vi "G-Vibro.vi"() -> ()   [LabVIEW 2016]
uses:
  <instrlib>/niScope/Controls/niScope trigger source.ctl
  <vilib>/Motion/FlexMotion/CustomControls/CustomControls.llb/AxisOrVectorSpace To Configure.flx
  <vilib>/Motion/FlexMotion/CustomControls/CustomControls.llb/AxisOrVectorSpaceControl To Control.flx
  <vilib>/event_ctls.llb/eventvkey.ctl
  <vilib>/Utility/file.llb/Write To Spreadsheet File (DBL).vi
  <vilib>/Motion/FlexMotion/FunctionsVIs/StartStopMotion.llb/Start Motion (8 axes).flx
  <vilib>/Motion/FlexMotion/FunctionsVIs/StartStopMotion.llb/Stop Motion (8 axes).flx
panel:
  out "Aceleration (pulse/s2)":i32
  out "Velocity (pulse/s)":i32
  in  "Power spectrum unit":string(combo)
  in  "Time unit":string(combo)
  in  "Highpass cut (kHz)":dbl=100.0
  in  "Center positioned":bool=TRUE
  out "Time (us)":dbl=-1000000.0
  out "Distance (mm)":dbl=-1480000.0
  out "Peak to peak":dbl
  in  "Lowpass filter":bool
  in  "Lowpass cut (kHz)":dbl=100.0
  out "Frequency Graph":cluster{"f0":dbl, "df":dbl, "magnitude":dbl[]}(graph)={"f0"=0.0, "df"=inf, "magnitude"=[]}
  out "z":dbl
  out "y":dbl=6.0
  out "x":dbl
  in  "Pulses":i32=20 min=1 max=100 step=1
  in  "Save to...":path=path "C:/Users/Vibro-PC/Desktop/Codigos em Labview/Data"
  in  "stop":bool
  in  "dz (mm)":dbl=1.0
  in  "Nz":i32=1 min=1 max=10000 step=1
  in  "dy (mm)":dbl=0.25
  in  "Ny":i32=56 min=1 max=10000 step=1
  in  "dx (mm)":dbl=0.25
  in  "Nx":i32=56 min=1 max=10000 step=1
  in  "Aceleration (mm/s2)":dbl=1000.0 min=50.0 max=1250.0 step=10.0
  out "Time Graph":waveform(dbl)(graph)={"t0"=timestamp(0 s since 1904-01-01), "dt"=1000000.0, "Y"=[]}
  in  "Enable Oscilloscope":bool
  in  "Move (mm)":dbl=6.0
  in  "Move Far":bool
  in  "Move Close":bool
  in  "Move Down":bool
  in  "Move Right":bool
  in  "Move Left":bool
  in  "Move Up":bool
  in  "Jog Far":bool
  in  "Jog Close":bool
  in  "Jog Down":bool
  in  "Jog Right":bool
  in  "Jog Left":bool
  in  "Jog Up":bool
  in  "Multiplier":dbl(slide)=0.10000000000000014 min=0.1 max=1.001 step=0.1 scale=0.1..1.0
  in  "Velocity (mm/s)":dbl=20.0 min=1.0 max=200.0 step=1.0
  in  "trigger level":dbl=2.0 caption="Level (V)" min=0.2 max=10.0 step=0.2 format="%.2f"
  in  "trigger source":T1="VAL_EXTERNAL" caption="Source"
  in  "Time (us)":dbl=2000.0 min=1.0 max=10000.0 step=1.0
  in  "Sample rate (MHz)":dbl=1.0 min=0.0 max=150.0 step=0.1 format="%.2f"
  in  "vertical offset":dbl caption="Offset (V)" min=-10.0 max=10.0 step=0.2 format="%.4f"
  in  "vertical range":dbl=2.0 caption="Vertical range (V)" min=0.0 max=20.0 format="%.2f"
  in  "# Channel":i32 min=0 max=1 step=1
  in  "Ajust Axis":bool
  in  "resource name":refnum<k15>="Dev1" caption="Source"
  # "Oscilloscope"
  # "Axis Stage"
  # "Channel Control"
  # "Temporal Control"
  # "Trigger Control"
  # "Status"
  # "Jog"
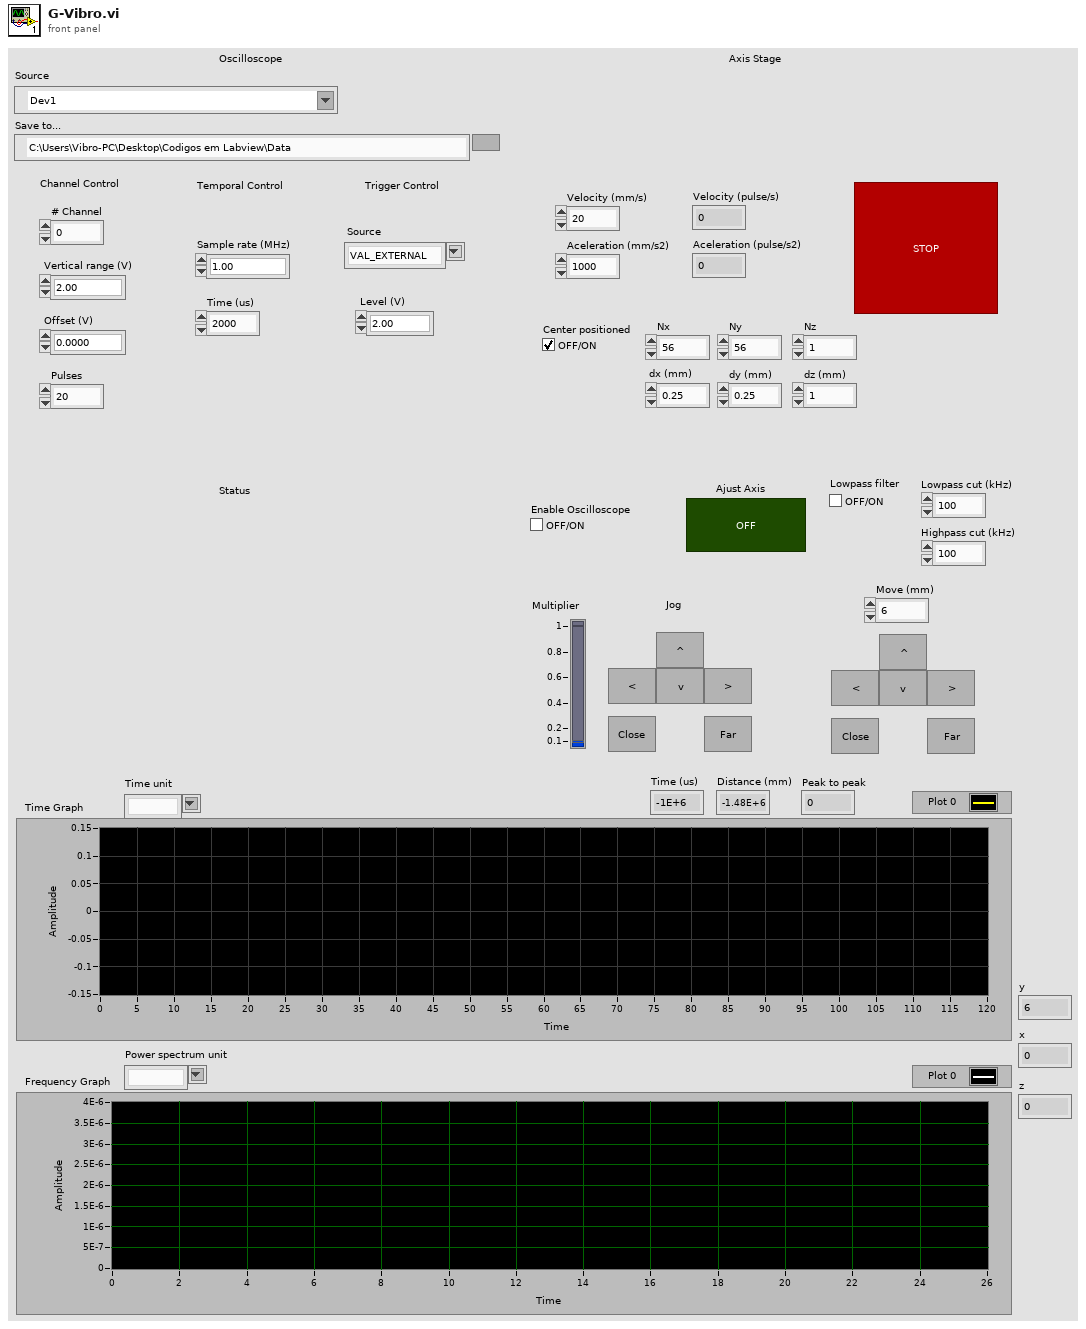
[diagram p1: front panel]
types:
  T1 = typedef "niScope trigger source.ctl" = string
  T2 = typedef "Board Id" = u8
  T3 = typedef "Bd Id Out" = u8
  T4 = enum16{"Absolute Position", "Relative Position", "Velocity", "Relative to Cap Pos", "Modulus Position", "Absolute Contouring", "Relative Contouring"}
  T5 = typedef "eventvkey.ctl" = enum16{"ASCII", "Enter", "Return", "Shift", "Ctrl", "Alt", "Cmd", "Opt", "Caps", "NumLock", "Clear", "Break", "Up", "Down", "Left", "Right", "Insert", "Delete", "Home", "End", "PageUp", "PageDown", "Escape", "Help", "Pause", "ScrollLock", "F1", "F2", "F3", "F4", "F5", "F6", "F7", "F8", "F9", "F10", "F11", "F12", "F13", "F14", "F15", "F16", "F17", "F18", "F19", "F20", "F21", "F22", "F23", "F24", "Play", "VolumeUp", "VolumeDown", "Mute", "Two Byte Char"}
  T6 = typedef "AxisOrVectorSpace To Configure.flx" = u16
  T7 = typedef "AxisOrVectorSpaceControl To Control.flx" = u16
  T8 = typedef "Resource Out (Enum).flx" = u16
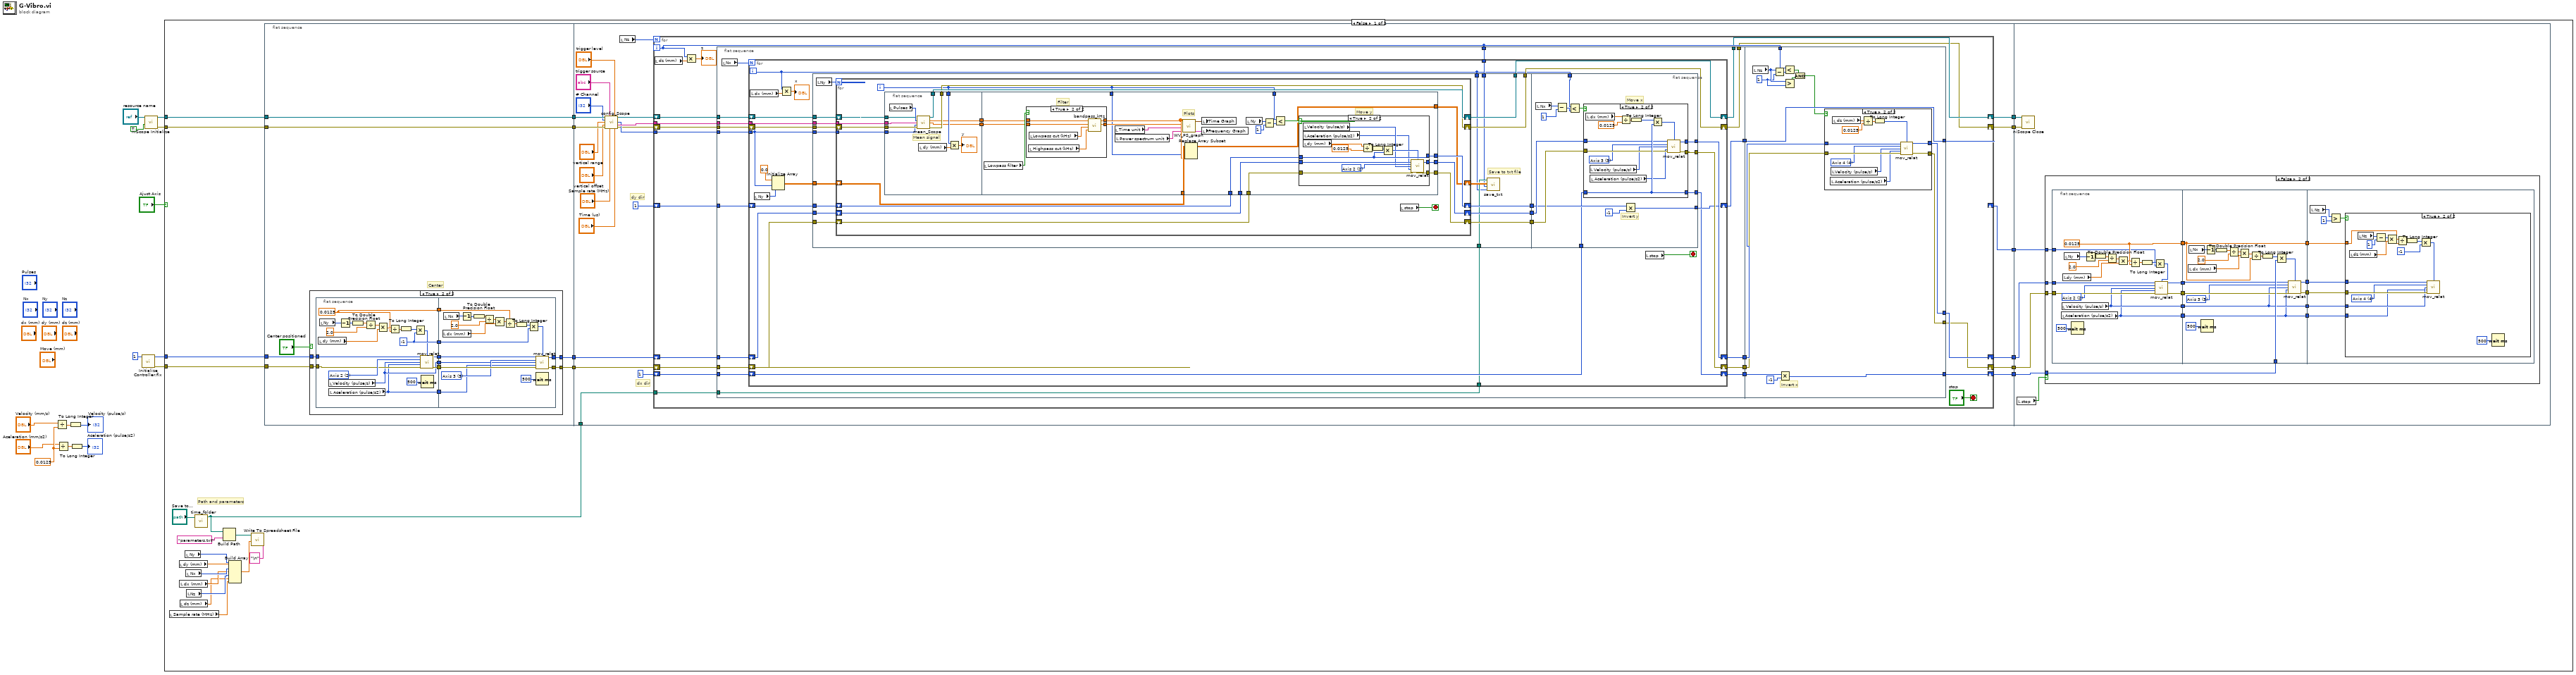
[diagram p0: block diagram]
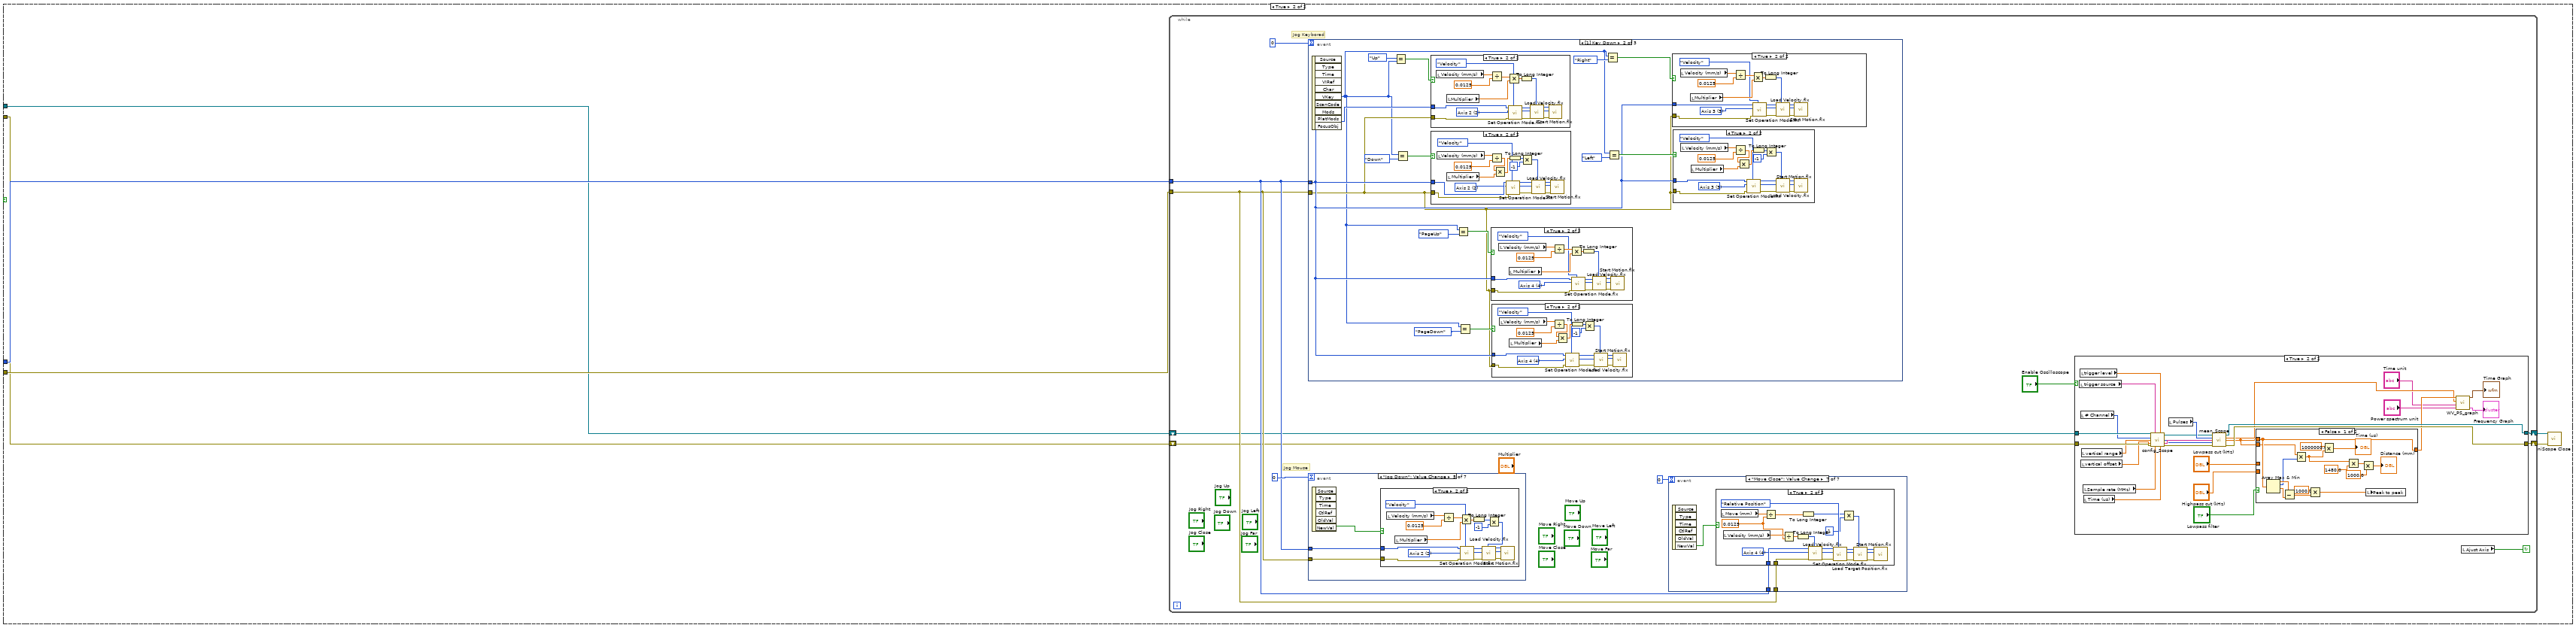
[diagram p9: hidden frame]
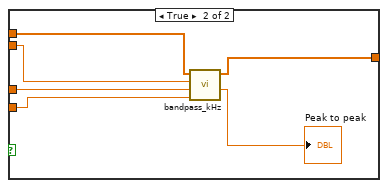
[diagram p11: hidden frame]
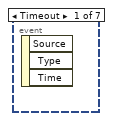
[diagram p12: hidden frame]
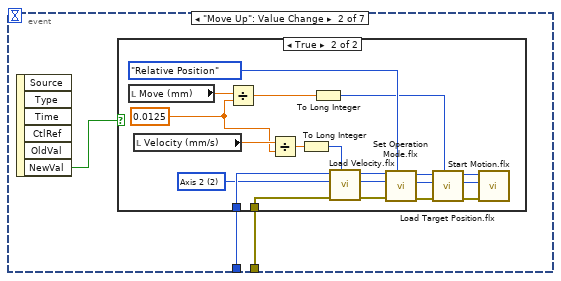
[diagram p13: hidden frame]
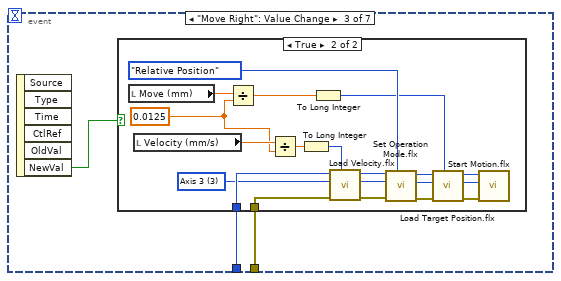
[diagram p15: hidden frame]
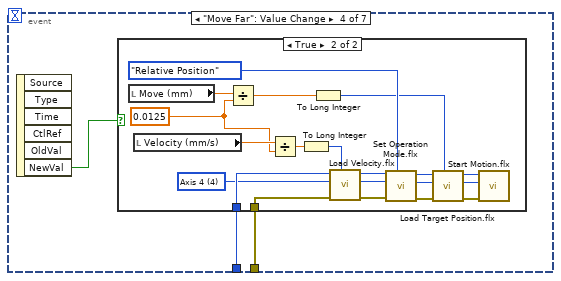
[diagram p17: hidden frame]
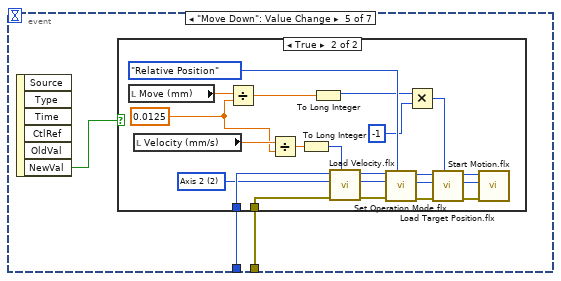
[diagram p19: hidden frame]
diagram:
  w6 = 0.0125
  n1 = Divide(x="Velocity (mm/s)", y=w6) -> (x/y=w4:dbl)
  n2 = Divide(x="Aceleration (mm/s2)", y=w6) -> (x/y=w3:dbl)
  n3 = To Long Integer(number=w4) -> (32bit integer=→"Velocity (pulse/s)":i32)
  n4 = To Long Integer(number=w3) -> (32bit integer=→"Aceleration (pulse/s2)":i32)
  n5 = call <vilib>:"Initialize Controller.flx"("Board ID"=T2 1) -> ("error out"=w9:errorcluster, "Bd ID Out"=w10:T3)  [unwired: 7 in]
  n6 = call <instrlib>:"niScope Initialize.vi"("resource name"="resource name", "reset device"=TRUE) -> ("instrument handle"=w13:refnum<k15>, "error out"=w12:errorcluster)  [unwired: 12 in]
  n7 = case shown="False" "Ajust Axis" {
    tunnel: w13 -> [w42 w432]
    tunnel: w12 -> [w41 w433]
    tunnel: w10 -> [w40 w435]
    tunnel: w9 -> [w39 w434]
    frame False {
      # "Path and parameters"
      n8 = local read "Sample rate (MHz)"() -> (w18:dbl)
      n9 = local read "dy (mm)"() -> (w23:dbl)
      n10 = local read "dx (mm)"() -> (w21:dbl)
      n11 = local read "dz (mm)"() -> (w19:dbl)
      n12 = local read "Ny"() -> (w24:i32)
      n13 = local read "Nx"() -> (w22:i32)
      n14 = local read "Nz"() -> (w20:i32)
      n15 = call "time_folder.vi"("base path"="Save to...") -> ("folder path"=w16:path)  [unwired: 9 in, 1 out]
      n16 = Build Path(base path=w16, name or relative path="parameters.txt") -> (appended path=w27:path)
      n17 = Build Array(w24, w23, w22, w21, w20, w19, w18) -> (w25:dbl[])
      n18 = call-poly <vilib>:"Write To Spreadsheet File.vi"("delimiter (\\t)"="\n", "1D data"=w25, "file path (dialog if empty)"=w27) -> ()  [unwired: 5 in, 1 out]
      n19 = flat-sequence {
        tunnel: w39 -> [w46]
        tunnel: w40 -> [w47]
        tunnel: w41 -> [w48]
        tunnel: w42 -> [w49]
        tunnel: [w49] -> w38
        tunnel: [w48] -> w37
        tunnel: [w45] -> w36
        tunnel: [w44] -> w35
        tunnel: w38 -> [w112]
        tunnel: w37 -> [w111]
        tunnel: w36 -> [w125]
        tunnel: w35 -> [w124]
        tunnel: [w121] -> w34
        tunnel: [w120] -> w33
        tunnel: [w119] -> w32
        tunnel: [w118] -> w31
        tunnel: [w117] -> w30
        tunnel: [w116] -> w29
        tunnel: w16 -> [w115]
        tunnel: w34 -> [w349]
        tunnel: w33 -> [w348]
        tunnel: w32 -> [w351]
        tunnel: w31 -> [w350]
        tunnel: w30 -> [w347]
        tunnel: w29 -> [w346]
        frame #0 {
          # "Center"
          n20 = case shown="True" "Center positioned" {
            tunnel: w47 -> [w51 w59]
            tunnel: w46 -> [w50 w58]
            tunnel: [w51 w53] -> w45
            tunnel: [w50 w52] -> w44
            frame False {
            }
            frame True {
              n21 = flat-sequence {
                tunnel: w59 -> [w67]
                tunnel: w58 -> [w66]
                tunnel: [w77] -> w61
                tunnel: [w75] -> w60
                tunnel: [w65] -> w57
                tunnel: [w64] -> w56
                tunnel: [w63] -> w55
                tunnel: [w62] -> w54
                tunnel: w61 -> [w97]
                tunnel: w60 -> [w95]
                tunnel: w57 -> [w89]
                tunnel: w56 -> [w88]
                tunnel: w55 -> [w86]
                tunnel: w54 -> [w85]
                tunnel: [w83] -> w53
                tunnel: [w82] -> w52
                frame #0 {
                  w75 = -1 ("y")
                  w77 = 0.0125
                  w68 = T6 2 items=["Axis 1"=1, "Axis 2"=2, "Axis 3"=3, "Axis 4"=4, "Axis 5"=5, "Axis 6"=6, "Axis 7"=7, "Axis 8"=8, "Vector Space 1"=17, "Vector Space 2"=18, "Vector Space 3"=19, "Vector Space 4"=20] ("Axis or Vector Space")
                  n22 = local read "dy (mm)"() -> (w80:dbl)
                  n23 = local read "Ny"() -> (w73:i32)
                  n24 = local read "Velocity (pulse/s)"() -> (w63:i32)
                  n25 = local read "Aceleration (pulse/s2)"() -> (w62:i32)
                  n26 = Decrement(x=w73) -> (x-1=w71:i32)
                  n27 = To Double Precision Float(number=w71) -> (double precision float=w72:dbl)
                  n28 = Divide(x=w72, y=2.0) -> (x/y=w81:dbl)
                  n29 = Multiply(x=w81, y=w80) -> (x*y=w79:dbl)
                  n30 = Divide(x=w79, y=w77) -> (x/y=w78:dbl)
                  n31 = To Long Integer(number=w78) -> (32bit integer=w76:i32)
                  n32 = Multiply(x=w76, y=w75) -> (x*y=w69:i32)
                  n33 = call "mov_relat.vi"("Board ID"=w67, "Target Position (0)"=w69, "Axis or Vector Space"=w68, "Velocity (10000)"=w63, "Acceleration (100000)"=w62, "error in (no error)"=w66) -> ("Bd ID Out"=w65:T3, "error out"=w64:errorcluster)  [unwired: 8 in]
                  n34 = Wait (ms)(milliseconds to wait=u32 500) -> ()  [unwired: 1 out]
                }
                frame #1 {
                  w87 = T6 3 items=["Axis 1"=1, "Axis 2"=2, "Axis 3"=3, "Axis 4"=4, "Axis 5"=5, "Axis 6"=6, "Axis 7"=7, "Axis 8"=8, "Vector Space 1"=17, "Vector Space 2"=18, "Vector Space 3"=19, "Vector Space 4"=20] ("Axis or Vector Space")
                  n35 = local read "dx (mm)"() -> (w98:dbl)
                  n36 = local read "Nx"() -> (w93:i32)
                  n37 = Decrement(x=w93) -> (x-1=w91:i32)
                  n38 = To Double Precision Float(number=w91) -> (double precision float=w92:dbl)
                  n39 = Divide(x=w92, y=2.0) -> (x/y=w101:dbl)
                  n40 = Multiply(x=w101, y=w98) -> (x*y=w100:dbl)
                  n41 = Divide(x=w100, y=w97) -> (x/y=w99:dbl)
                  n42 = To Long Integer(number=w99) -> (32bit integer=w96:i32)
                  n43 = Multiply(x=w96, y=w95) -> (x*y=w84:i32)
                  n44 = Wait (ms)(milliseconds to wait=u32 500) -> ()  [unwired: 1 out]
                  n45 = call "mov_relat.vi"("Board ID"=w89, "Target Position (0)"=w84, "Axis or Vector Space"=w87, "Velocity (10000)"=w86, "Acceleration (100000)"=w85, "error in (no error)"=w88) -> ("Bd ID Out"=w83:T3, "error out"=w82:errorcluster)  [unwired: 8 in]
                }
              }
            }
          }
        }
        frame #1 {
          # "dx dir"
          # "dy dir"
          n46 = call "config_Scope.vi"("instrument handle"=w112, "trigger source"="trigger source", "trigger level"="trigger level", "Channel"="# Channel", "vertical range"="vertical range", "vertical offset"="vertical offset", "error in"=w111, "Frequency(MHz)"="Sample rate (MHz)", "Time(us)"="Time (us)") -> ("instrument handle out"=w103:refnum<k15>, "Record length"=w113:i32, "Channel out"=w114:string, "error out"=w102:errorcluster)  [unwired: 3 in]
          n47 = local read "Nz"() -> (w126:i32)
          n48 = for {
            N: w126 -> [_]
            tunnel: w114 -> [w146]
            shift-right: [w127] -> w118
            shift-left: w102 -> [w147]
            shift-right: [w128] -> w119
            shift-left: w103 -> [w148]
            shift-right: [w135] -> w121
            shift-left: w125 -> [w145]
            shift-right: [w134] -> w120
            shift-left: w124 -> [w144]
            shift-right: [w142] -> w117
            shift-left: 1 -> [w143]
            shift-right: [w136] -> w116
            shift-left: 1 -> [w141]
            tunnel: w113 -> [w133]
            tunnel: w115 -> [w132]
            i -> [w129]
            stop <- "stop" stop-if-true
            n49 = local read "dz (mm)"() -> (w130:dbl)
            n50 = Multiply(x=w129, y=w130) -> (x*y=→"z":dbl)
            n51 = flat-sequence {
              tunnel: w148 -> [w165]
              tunnel: w147 -> [w164]
              tunnel: w146 -> [w163]
              tunnel: w145 -> [w162]
              tunnel: w144 -> [w161]
              tunnel: w143 -> [w158]
              tunnel: w141 -> [w156]
              tunnel: [w160] -> w140
              tunnel: [w159] -> w139
              tunnel: [w157] -> w138
              tunnel: [w155] -> w137
              tunnel: w133 -> [w154]
              tunnel: w132 -> [w153]
              tunnel: w129 -> [w152]
              tunnel: [w151] -> w128
              tunnel: [w150] -> w127
              tunnel: [w328] -> w136
              tunnel: [w331] -> w142
              tunnel: w140 -> [w320]
              tunnel: w139 -> [w319]
              tunnel: w138 -> [w331]
              tunnel: w137 -> [w329]
              tunnel: w129 -> [w326]
              tunnel: [w318] -> w135
              tunnel: [w317] -> w134
              frame #0 {
                n52 = local read "Nx"() -> (w166:i32)
                n53 = for {
                  N: w166 -> [_]
                  shift-right: [w184] -> w151
                  shift-left: w165 -> [w191]
                  tunnel: w163 -> [w189]
                  shift-right: [w183] -> w150
                  shift-left: w164 -> [w190]
                  shift-right: [w182] -> w160
                  shift-left: w162 -> [w188]
                  shift-right: [w181] -> w159
                  shift-left: w161 -> [w187]
                  shift-right: [w178] -> w157
                  shift-left: w158 -> [w180]
                  shift-right: [w176] -> w155
                  shift-left: w156 -> [w177]
                  tunnel: w154 -> [w171]
                  tunnel: w153 -> [w167]
                  tunnel: w152 -> [w172]
                  i -> [w168]
                  stop <- w192 stop-if-true
                  n54 = local read "dx (mm)"() -> (w170:dbl)
                  n55 = local read "Ny"() -> (w174:i32)
                  n56 = Initialize Array(0.0 ("element"), w171, w174) -> (w173:dbl[][])
                  n57 = Multiply(x=w168, y=w170) -> (x*y=→"x":dbl)
                  n58 = flat-sequence {
                    tunnel: w191 -> [w209]
                    tunnel: w190 -> [w208]
                    tunnel: w189 -> [w207]
                    tunnel: w188 -> [w206]
                    tunnel: w187 -> [w205]
                    tunnel: [w204] -> w186
                    tunnel: [w203] -> w185
                    tunnel: [w202] -> w184
                    tunnel: [w201] -> w183
                    tunnel: w180 -> [w200]
                    tunnel: [w199] -> w179
                    tunnel: w173 -> [w198]
                    tunnel: w167 -> [w195]
                    tunnel: w168 -> [w193]
                    tunnel: w172 -> [w194]
                    tunnel: w171 -> [w197]
                    tunnel: w186 -> [w300]
                    tunnel: w185 -> [w299]
                    tunnel: w168 -> [w297]
                    tunnel: [w296] -> w182
                    tunnel: [w295] -> w181
                    tunnel: w179 -> [w294]
                    tunnel: [w292] -> w178
                    tunnel: w177 -> [w288]
                    tunnel: [w287] -> w176
                    frame #0 {
                      # "Save to txt file"
                      n59 = local read "Ny"() -> (w210:i32)
                      n60 = for {
                        N: w210 -> [_]
                        shift-right: [w214] -> w202
                        shift-left: w209 -> [w225]
                        tunnel: w207 -> [w226]
                        shift-right: [w213] -> w201
                        shift-left: w208 -> [w227]
                        shift-right: [w222] -> w204
                        shift-left: w206 -> [w224]
                        shift-right: [w221] -> w203
                        shift-left: w205 -> [w223]
                        shift-right: [w220] -> w199
                        shift-left: w200 -> [w218]
                        shift-right: [w216] -> w196
                        shift-left: w198 -> [w219]
                        tunnel: w197 -> [w217]
                        i -> [w211]
                        stop <- w228 stop-if-true
                        n61 = flat-sequence {
                          tunnel: w227 -> [w231]
                          tunnel: w226 -> [w229]
                          tunnel: w225 -> [w232]
                          tunnel: w211 -> [w240]
                          tunnel: w217 -> [w230]
                          tunnel: [w234] -> w215
                          tunnel: [w237] -> w214
                          tunnel: [w236] -> w213
                          tunnel: [w235] -> w212
                          tunnel: w224 -> [w263]
                          tunnel: w223 -> [w262]
                          tunnel: [w261] -> w222
                          tunnel: [w260] -> w221
                          tunnel: w211 -> [w251]
                          tunnel: [w258] -> w220
                          tunnel: w219 -> [w253]
                          tunnel: w218 -> [w254]
                          tunnel: [w252] -> w216
                          tunnel: w215 -> [w247]
                          tunnel: w212 -> [w249]
                          tunnel: w211 -> [w241]
                          frame #0 {
                            # "Mean signal"
                            n62 = local read "Pulses"() -> (w233:i32)
                            n63 = call "mean_Scope.vi"("instrument handle in"=w232, "pulses"=w233, "channels"=w229, "record length"=w230, "error in"=w231) -> ("instrument handle out"=w237:refnum<k15>, "signal out"=w235:dbl[], "dt"=w234:dbl, "error out"=w236:errorcluster)  [unwired: 7 in]
                            n64 = local read "dy (mm)"() -> (w238:dbl)
                            n65 = Multiply(x=w240, y=w238) -> (x*y=→"y":dbl)
                          }
                          frame #1 {
                            # "Move y"
                            # "Plots"
                            # "Filter"
                            n66 = local read "Lowpass filter"() -> (w250:bool)
                            n67 = case shown="True" w250 {
                              tunnel: w249 -> [w265 w270]
                              tunnel: [w265 w269] -> w248
                              tunnel: w247 -> [w264 w266]
                              tunnel: [w264 w266] -> w242
                              frame False {
                              }
                              frame True {
                                n68 = local read "Highpass cut (kHz)"() -> (w267:dbl)
                                n69 = local read "Lowpass cut (kHz)"() -> (w268:dbl)
                                n70 = call "bandpass_kHz.vi"("Highpass cut (kHz)"=w267, "Lowpass cut (kHz)"=w268, "dt"=w266, "Signal in"=w270) -> ("Signal out"=w269:dbl[])  [unwired: 6 in, 1 out]
                              }
                            }
                            n71 = local read "Time unit"() -> (w246:string)
                            n72 = local read "Power spectrum unit"() -> (w245:string)
                            n73 = call "WV_PS_graph.vi"("Power spectrum unit"=w245, "Time unit"=w246, "dt"=w242, "Signal in"=w248) -> ("Power Spectrum / PSD"=w244:cluster{"f0":dbl, "df":dbl, "magnitude":dbl[]}, "output waveform"=w243:waveform(dbl))  [unwired: 6 in]
                            n74 = Replace Array Subset(array=w253, new element=w248, index (col)=w241) -> (w252:dbl[][])  [unwired: 1 in]
                            n75 = local write "Time Graph"(w243) -> ()
                            n76 = local write "Frequency Graph"(w244) -> ()
                            n77 = local read "Ny"() -> (w257:i32)
                            n78 = Subtract(x=w257, y=1) -> (x-y=w255:i32)
                            n79 = Less?(x=w251, y=w255) -> (x < y?=w259:bool)
                            n80 = case shown="True" w259 {
                              tunnel: w263 -> [w272 w281]
                              tunnel: w262 -> [w273 w280]
                              tunnel: [w272 w277] -> w261
                              tunnel: [w273 w276] -> w260
                              tunnel: w254 -> [w271 w282]
                              tunnel: [w271 w282] -> w258
                              frame False {
                              }
                              frame True {
                                w279 = T6 2 items=["Axis 1"=1, "Axis 2"=2, "Axis 3"=3, "Axis 4"=4, "Axis 5"=5, "Axis 6"=6, "Axis 7"=7, "Axis 8"=8, "Vector Space 1"=17, "Vector Space 2"=18, "Vector Space 3"=19, "Vector Space 4"=20] ("Axis or Vector Space")
                                n81 = local read "Velocity (pulse/s)"() -> (w275:i32)
                                n82 = local read "Aceleration (pulse/s2)"() -> (w274:i32)
                                n83 = local read "dy (mm)"() -> (w286:dbl)
                                n84 = Divide(x=w286, y=0.0125) -> (x/y=w284:dbl)
                                n85 = To Long Integer(number=w284) -> (32bit integer=w283:i32)
                                n86 = Multiply(x=w283, y=w282) -> (x*y=w278:i32)
                                n87 = call "mov_relat.vi"("Board ID"=w281, "Target Position (0)"=w278, "Axis or Vector Space"=w279, "Velocity (10000)"=w275, "Acceleration (100000)"=w274, "error in (no error)"=w280) -> ("Bd ID Out"=w277:T3, "error out"=w276:errorcluster)  [unwired: 8 in]
                              }
                            }
                          }
                        }
                        n88 = local read "stop"() -> (w228:bool)
                      }
                      n89 = call "save_txt.vi"("x"=w193, "z"=w194, "Data"=w196, "base path"=w195) -> ()  [unwired: 8 in]
                    }
                    frame #1 {
                      # "Move x"
                      # "Invert y"
                      n90 = local read "Nx"() -> (w291:i32)
                      n91 = Subtract(x=w291, y=1) -> (x-y=w289:i32)
                      n92 = Less?(x=w297, y=w289) -> (x < y?=w298:bool)
                      n93 = case shown="True" w298 {
                        tunnel: w300 -> [w301 w311]
                        tunnel: w299 -> [w303 w310]
                        tunnel: [w301 w309] -> w296
                        tunnel: [w303 w308] -> w295
                        tunnel: w288 -> [w302 w312]
                        tunnel: [w302 w312] -> w287
                        frame False {
                        }
                        frame True {
                          w307 = T6 3 items=["Axis 1"=1, "Axis 2"=2, "Axis 3"=3, "Axis 4"=4, "Axis 5"=5, "Axis 6"=6, "Axis 7"=7, "Axis 8"=8, "Vector Space 1"=17, "Vector Space 2"=18, "Vector Space 3"=19, "Vector Space 4"=20] ("Axis or Vector Space")
                          n94 = local read "dx (mm)"() -> (w314:dbl)
                          n95 = local read "Velocity (pulse/s)"() -> (w306:i32)
                          n96 = local read "Aceleration (pulse/s2)"() -> (w305:i32)
                          n97 = Divide(x=w314, y=0.0125) -> (x/y=w315:dbl)
                          n98 = To Long Integer(number=w315) -> (32bit integer=w313:i32)
                          n99 = Multiply(x=w313, y=w312) -> (x*y=w304:i32)
                          n100 = call "mov_relat.vi"("Board ID"=w311, "Target Position (0)"=w304, "Axis or Vector Space"=w307, "Velocity (10000)"=w306, "Acceleration (100000)"=w305, "error in (no error)"=w310) -> ("Bd ID Out"=w309:T3, "error out"=w308:errorcluster)  [unwired: 8 in]
                        }
                      }
                      n101 = Multiply(x=w294, y=-1) -> (x*y=w292:i32)
                    }
                  }
                  n102 = local read "stop"() -> (w192:bool)
                }
              }
              frame #1 {
                w324 = 1 ("y")
                # "Invert x"
                n103 = local read "Nz"() -> (w325:i32)
                n104 = Subtract(x=w325, y=w324) -> (x-y=w327:i32)
                n105 = Multiply(x=w329, y=-1) -> (x*y=w328:i32)
                n106 = Less?(x=w326, y=w327) -> (x < y?=w323:bool)
                n107 = Greater?(x=w325, y=w324) -> (0:w322:bool)
                n108 = And(x=w323, y=w322) -> (x .and. y?=w321:bool)
                n109 = case shown="True" w321 {
                  tunnel: w320 -> [w333 w341]
                  tunnel: w319 -> [w332 w340]
                  tunnel: [w333 w335] -> w318
                  tunnel: [w332 w334] -> w317
                  frame False {
                  }
                  frame True {
                    w339 = T6 4 items=["Axis 1"=1, "Axis 2"=2, "Axis 3"=3, "Axis 4"=4, "Axis 5"=5, "Axis 6"=6, "Axis 7"=7, "Axis 8"=8, "Vector Space 1"=17, "Vector Space 2"=18, "Vector Space 3"=19, "Vector Space 4"=20] ("Axis or Vector Space")
                    n110 = local read "Aceleration (pulse/s2)"() -> (w337:i32)
                    n111 = local read "Velocity (pulse/s)"() -> (w338:i32)
                    n112 = local read "dz (mm)"() -> (w342:dbl)
                    n113 = Divide(x=w342, y=0.0125) -> (x/y=w343:dbl)
                    n114 = To Long Integer(number=w343) -> (32bit integer=w336:i32)
                    n115 = call "mov_relat.vi"("Board ID"=w341, "Target Position (0)"=w336, "Axis or Vector Space"=w339, "Velocity (10000)"=w338, "Acceleration (100000)"=w337, "error in (no error)"=w340) -> ("Bd ID Out"=w335:T3, "error out"=w334:errorcluster)  [unwired: 8 in]
                  }
                }
              }
            }
          }
        }
        frame #2 {
          n116 = local read "stop"() -> (w345:bool)
          n117 = call <instrlib>:"niScope Close.vi"("instrument handle"=w351, "error in"=w350) -> ()  [unwired: 13 in, 1 out]
          n118 = case shown="False" w345 {
            tunnel: w349 -> [_ w363]
            tunnel: w348 -> [_ w362]
            tunnel: w347 -> [_ w361]
            tunnel: w346 -> [_ w360]
            frame True {
            }
            frame False {
              n119 = flat-sequence {
                tunnel: w363 -> [w373]
                tunnel: w362 -> [w372]
                tunnel: [w381] -> w365
                tunnel: w361 -> [w378]
                tunnel: [w369] -> w359
                tunnel: [w368] -> w358
                tunnel: [w367] -> w357
                tunnel: [w366] -> w356
                tunnel: w365 -> [w398]
                tunnel: w360 -> [w399]
                tunnel: [w398] -> w364
                tunnel: w359 -> [w392]
                tunnel: w358 -> [w391]
                tunnel: w357 -> [w387]
                tunnel: w356 -> [w386]
                tunnel: [w389] -> w355
                tunnel: [w388] -> w354
                tunnel: [w387] -> w353
                tunnel: [w386] -> w352
                tunnel: w364 -> [w413]
                tunnel: w355 -> [w409]
                tunnel: w354 -> [w408]
                tunnel: w353 -> [w407]
                tunnel: w352 -> [w406]
                frame #0 {
                  w381 = 0.0125
                  w371 = T6 2 items=["Axis 1"=1, "Axis 2"=2, "Axis 3"=3, "Axis 4"=4, "Axis 5"=5, "Axis 6"=6, "Axis 7"=7, "Axis 8"=8, "Vector Space 1"=17, "Vector Space 2"=18, "Vector Space 3"=19, "Vector Space 4"=20] ("Axis or Vector Space")
                  n120 = local read "Aceleration (pulse/s2)"() -> (w366:i32)
                  n121 = local read "Velocity (pulse/s)"() -> (w367:i32)
                  n122 = local read "dy (mm)"() -> (w384:dbl)
                  n123 = local read "Ny"() -> (w377:i32)
                  n124 = Wait (ms)(milliseconds to wait=u32 500) -> ()  [unwired: 1 out]
                  n125 = Decrement(x=w377) -> (x-1=w375:i32)
                  n126 = To Double Precision Float(number=w375) -> (double precision float=w376:dbl)
                  n127 = Divide(x=w376, y=2.0) -> (x/y=w385:dbl)
                  n128 = Multiply(x=w385, y=w384) -> (x*y=w383:dbl)
                  n129 = Divide(x=w383, y=w381) -> (x/y=w382:dbl)
                  n130 = To Long Integer(number=w382) -> (32bit integer=w380:i32)
                  n131 = Multiply(x=w380, y=w378) -> (x*y=w370:i32)
                  n132 = call "mov_relat.vi"("Board ID"=w373, "Target Position (0)"=w370, "Axis or Vector Space"=w371, "Velocity (10000)"=w367, "Acceleration (100000)"=w366, "error in (no error)"=w372) -> ("Bd ID Out"=w369:T3, "error out"=w368:errorcluster)  [unwired: 8 in]
                }
                frame #1 {
                  w390 = T6 3 items=["Axis 1"=1, "Axis 2"=2, "Axis 3"=3, "Axis 4"=4, "Axis 5"=5, "Axis 6"=6, "Axis 7"=7, "Axis 8"=8, "Vector Space 1"=17, "Vector Space 2"=18, "Vector Space 3"=19, "Vector Space 4"=20] ("Axis or Vector Space")
                  n133 = local read "dx (mm)"() -> (w402:dbl)
                  n134 = local read "Nx"() -> (w397:i32)
                  n135 = Wait (ms)(milliseconds to wait=u32 500) -> ()  [unwired: 1 out]
                  n136 = Decrement(x=w397) -> (x-1=w396:i32)
                  n137 = To Double Precision Float(number=w396) -> (double precision float=w395:dbl)
                  n138 = Divide(x=w395, y=2.0) -> (x/y=w405:dbl)
                  n139 = Multiply(x=w405, y=w402) -> (x*y=w404:dbl)
                  n140 = Divide(x=w404, y=w398) -> (x/y=w403:dbl)
                  n141 = To Long Integer(number=w403) -> (32bit integer=w401:i32)
                  n142 = Multiply(x=w401, y=w399) -> (x*y=w393:i32)
                  n143 = call "mov_relat.vi"("Board ID"=w392, "Target Position (0)"=w393, "Axis or Vector Space"=w390, "Velocity (10000)"=w387, "Acceleration (100000)"=w386, "error in (no error)"=w391) -> ("Bd ID Out"=w389:T3, "error out"=w388:errorcluster)  [unwired: 8 in]
                }
                frame #2 {
                  n144 = local read "Nz"() -> (w411:i32)
                  n145 = Greater?(x=w411, y=1) -> (0:w412:bool)
                  n146 = case shown="True" w412 {
                    tunnel: w413 -> [_ w424]
                    tunnel: w409 -> [_ w419]
                    tunnel: w408 -> [_ w418]
                    tunnel: w407 -> [_ w415]
                    tunnel: w406 -> [_ w414]
                    frame False {
                    }
                    frame True {
                      w416 = T6 4 items=["Axis 1"=1, "Axis 2"=2, "Axis 3"=3, "Axis 4"=4, "Axis 5"=5, "Axis 6"=6, "Axis 7"=7, "Axis 8"=8, "Vector Space 1"=17, "Vector Space 2"=18, "Vector Space 3"=19, "Vector Space 4"=20] ("Axis or Vector Space")
                      n147 = local read "dz (mm)"() -> (w425:dbl)
                      n148 = local read "Nz"() -> (w422:i32)
                      n149 = Subtract(x=w422, y=1) -> (x-y=w421:i32)
                      n150 = Multiply(x=w421, y=w425) -> (x*y=w429:dbl)
                      n151 = Divide(x=w429, y=w424) -> (x/y=w428:dbl)
                      n152 = To Long Integer(number=w428) -> (32bit integer=w427:i32)
                      n153 = Multiply(x=w427, y=-1) -> (x*y=w417:i32)
                      n154 = call "mov_relat.vi"("Board ID"=w419, "Target Position (0)"=w417, "Axis or Vector Space"=w416, "Velocity (10000)"=w415, "Acceleration (100000)"=w414, "error in (no error)"=w418) -> ()  [unwired: 8 in, 2 out]
                      n155 = Wait (ms)(milliseconds to wait=u32 500) -> ()  [unwired: 1 out]
                    }
                  }
                }
              }
            }
          }
        }
      }
    }
    frame True {
      n156 = while {
        tunnel: w435 -> [w443]
        tunnel: w434 -> [w442]
        shift-right: [w438] -> w431
        shift-left: w432 -> [w439]
        shift-right: [w437] -> w430
        shift-left: w433 -> [w440]
        stop <- w446 continue-if-true
        # "Jog Mouse"
        # "Jog Keyborad"
        n157 = event shown="[1] Key Down" {
          selector: _ -> [_ _ _]
          dyn-events: _ -> [_ _ _]
          timeout: 0 -> [_ _ _]
          tunnel: w443 -> [_ w642 w757]
          tunnel: w442 -> [_ w641 w759]
          event Timeout {
            n158 = event-data() -> ()  [unwired: 1 in, 3 out]
          }
          event Key Down {
            n159 = event-data() -> ("VKey"=w640:T5)  [unwired: 1 in, 9 out]
            n160 = Equal?(x=eventvkey."Up" ("VKey"), y=w640) -> (x = y?=w653:bool)
            n161 = Equal?(x=w640, y=eventvkey."Down" ("VKey")) -> (x = y?=w652:bool)
            n162 = case shown="True" w653 {
              tunnel: w642 -> [_ w746]
              tunnel: w641 -> [_ w745]
              frame False {
              }
              frame True {
                w747 = T7 2 items=["Axis Control"=0, "Axis 1"=1, "Axis 2"=2, "Axis 3"=3, "Axis 4"=4, "Axis 5"=5, "Axis 6"=6, "Axis 7"=7, "Axis 8"=8, "Vector Space Control"=16, "Vector Space 1"=17, "Vector Space 2"=18, "Vector Space 3"=19, "Vector Space 4"=20] ("Axis or Vector Space")
                n163 = local read "Velocity (mm/s)"() -> (w753:dbl)
                n164 = local read "Multiplier"() -> (w748:dbl)
                n165 = Divide(x=w753, y=0.0125) -> (x/y=w750:dbl)
                n166 = Multiply(x=w750, y=w748) -> (x*y=w749:dbl)
                n167 = call <vilib>:"Set Operation Mode.flx"("Position Mode (Absolute)"=T4."Velocity", "error in (no error)"=w745, "Axis or Vector Space"=w747, "Board ID"=w746) -> ("error out"=w742:errorcluster, "Resource Output"=w743:T8, "Bd ID Out"=w744:T3)  [unwired: 2 in]
                n168 = To Long Integer(number=w749) -> (32bit integer=w751:i32)
                n169 = call <vilib>:"Load Velocity.flx"("Velocity (10000)"=w751, "error in (no error)"=w742, "Axis or Vector Space"=w743, "Board ID"=w744) -> ("error out"=w754:errorcluster, "Resource Output"=w755:T8, "Bd ID Out"=w756:T3)  [unwired: 3 in]
                n170 = call-poly <vilib>:"Start Motion.flx"("error in (no error)"=w754, "Axis or Vector Space"=w755, "Board ID"=w756) -> ()  [unwired: 3 in, 3 out]
              }
            }
            n171 = case shown="True" w652 {
              tunnel: w642 -> [_ w729]
              tunnel: w641 -> [_ w728]
              frame False {
              }
              frame True {
                w727 = T7 2 items=["Axis Control"=0, "Axis 1"=1, "Axis 2"=2, "Axis 3"=3, "Axis 4"=4, "Axis 5"=5, "Axis 6"=6, "Axis 7"=7, "Axis 8"=8, "Vector Space Control"=16, "Vector Space 1"=17, "Vector Space 2"=18, "Vector Space 3"=19, "Vector Space 4"=20] ("Axis or Vector Space")
                n172 = local read "Velocity (mm/s)"() -> (w736:dbl)
                n173 = local read "Multiplier"() -> (w730:dbl)
                n174 = Divide(x=w736, y=0.0125) -> (x/y=w732:dbl)
                n175 = Multiply(x=w732, y=w730) -> (x*y=w731:dbl)
                n176 = call <vilib>:"Set Operation Mode.flx"("Position Mode (Absolute)"=T4."Velocity", "error in (no error)"=w728, "Axis or Vector Space"=w727, "Board ID"=w729) -> ("error out"=w724:errorcluster, "Resource Output"=w725:T8, "Bd ID Out"=w726:T3)  [unwired: 2 in]
                n177 = To Long Integer(number=w731) -> (32bit integer=w735:i32)
                n178 = Multiply(x=w735, y=-1) -> (x*y=w733:i32)
                n179 = call <vilib>:"Load Velocity.flx"("Velocity (10000)"=w733, "error in (no error)"=w724, "Axis or Vector Space"=w725, "Board ID"=w726) -> ("error out"=w738:errorcluster, "Resource Output"=w739:T8, "Bd ID Out"=w740:T3)  [unwired: 3 in]
                n180 = call-poly <vilib>:"Start Motion.flx"("error in (no error)"=w738, "Axis or Vector Space"=w739, "Board ID"=w740) -> ()  [unwired: 3 in, 3 out]
              }
            }
            n181 = Equal?(x=w640, y=eventvkey."PageUp" ("VKey")) -> (x = y?=w646:bool)
            n182 = Equal?(x=w640, y=eventvkey."PageDown" ("VKey")) -> (x = y?=w645:bool)
            n183 = case shown="True" w646 {
              tunnel: w642 -> [_ w678]
              tunnel: w641 -> [_ w677]
              frame False {
              }
              frame True {
                w679 = T7 4 items=["Axis Control"=0, "Axis 1"=1, "Axis 2"=2, "Axis 3"=3, "Axis 4"=4, "Axis 5"=5, "Axis 6"=6, "Axis 7"=7, "Axis 8"=8, "Vector Space Control"=16, "Vector Space 1"=17, "Vector Space 2"=18, "Vector Space 3"=19, "Vector Space 4"=20] ("Axis or Vector Space")
                n184 = local read "Velocity (mm/s)"() -> (w685:dbl)
                n185 = local read "Multiplier"() -> (w680:dbl)
                n186 = Divide(x=w685, y=0.0125) -> (x/y=w682:dbl)
                n187 = Multiply(x=w682, y=w680) -> (x*y=w681:dbl)
                n188 = call <vilib>:"Set Operation Mode.flx"("Position Mode (Absolute)"=T4."Velocity", "error in (no error)"=w677, "Axis or Vector Space"=w679, "Board ID"=w678) -> ("error out"=w675:errorcluster, "Resource Output"=w674:T8, "Bd ID Out"=w676:T3)  [unwired: 2 in]
                n189 = To Long Integer(number=w681) -> (32bit integer=w683:i32)
                n190 = call <vilib>:"Load Velocity.flx"("Velocity (10000)"=w683, "error in (no error)"=w675, "Axis or Vector Space"=w674, "Board ID"=w676) -> ("error out"=w686:errorcluster, "Resource Output"=w687:T8, "Bd ID Out"=w688:T3)  [unwired: 3 in]
                n191 = call-poly <vilib>:"Start Motion.flx"("error in (no error)"=w686, "Axis or Vector Space"=w687, "Board ID"=w688) -> ()  [unwired: 3 in, 3 out]
              }
            }
            n192 = case shown="True" w645 {
              tunnel: w642 -> [_ w661]
              tunnel: w641 -> [_ w660]
              frame False {
              }
              frame True {
                w659 = T7 4 items=["Axis Control"=0, "Axis 1"=1, "Axis 2"=2, "Axis 3"=3, "Axis 4"=4, "Axis 5"=5, "Axis 6"=6, "Axis 7"=7, "Axis 8"=8, "Vector Space Control"=16, "Vector Space 1"=17, "Vector Space 2"=18, "Vector Space 3"=19, "Vector Space 4"=20] ("Axis or Vector Space")
                n193 = local read "Velocity (mm/s)"() -> (w668:dbl)
                n194 = local read "Multiplier"() -> (w662:dbl)
                n195 = Divide(x=w668, y=0.0125) -> (x/y=w664:dbl)
                n196 = Multiply(x=w664, y=w662) -> (x*y=w663:dbl)
                n197 = call <vilib>:"Set Operation Mode.flx"("Position Mode (Absolute)"=T4."Velocity", "error in (no error)"=w660, "Axis or Vector Space"=w659, "Board ID"=w661) -> ("error out"=w656:errorcluster, "Resource Output"=w658:T8, "Bd ID Out"=w657:T3)  [unwired: 2 in]
                n198 = To Long Integer(number=w663) -> (32bit integer=w667:i32)
                n199 = Multiply(x=w667, y=-1) -> (x*y=w665:i32)
                n200 = call <vilib>:"Load Velocity.flx"("Velocity (10000)"=w665, "error in (no error)"=w656, "Axis or Vector Space"=w658, "Board ID"=w657) -> ("error out"=w670:errorcluster, "Resource Output"=w671:T8, "Bd ID Out"=w672:T3)  [unwired: 3 in]
                n201 = call-poly <vilib>:"Start Motion.flx"("error in (no error)"=w670, "Axis or Vector Space"=w671, "Board ID"=w672) -> ()  [unwired: 3 in, 3 out]
              }
            }
            n202 = Equal?(x=w640, y=eventvkey."Right" ("VKey")) -> (x = y?=w650:bool)
            n203 = Equal?(x=w640, y=eventvkey."Left" ("VKey")) -> (x = y?=w649:bool)
            n204 = case shown="True" w650 {
              tunnel: w642 -> [_ w712]
              tunnel: w641 -> [_ w711]
              frame False {
              }
              frame True {
                w713 = T7 3 items=["Axis Control"=0, "Axis 1"=1, "Axis 2"=2, "Axis 3"=3, "Axis 4"=4, "Axis 5"=5, "Axis 6"=6, "Axis 7"=7, "Axis 8"=8, "Vector Space Control"=16, "Vector Space 1"=17, "Vector Space 2"=18, "Vector Space 3"=19, "Vector Space 4"=20] ("Axis or Vector Space")
                n205 = local read "Velocity (mm/s)"() -> (w719:dbl)
                n206 = local read "Multiplier"() -> (w714:dbl)
                n207 = Divide(x=w719, y=0.0125) -> (x/y=w716:dbl)
                n208 = Multiply(x=w716, y=w714) -> (x*y=w715:dbl)
                n209 = call <vilib>:"Set Operation Mode.flx"("Position Mode (Absolute)"=T4."Velocity", "error in (no error)"=w711, "Axis or Vector Space"=w713, "Board ID"=w712) -> ("error out"=w709:errorcluster, "Resource Output"=w708:T8, "Bd ID Out"=w710:T3)  [unwired: 2 in]
                n210 = To Long Integer(number=w715) -> (32bit integer=w717:i32)
                n211 = call <vilib>:"Load Velocity.flx"("Velocity (10000)"=w717, "error in (no error)"=w709, "Axis or Vector Space"=w708, "Board ID"=w710) -> ("error out"=w720:errorcluster, "Resource Output"=w721:T8, "Bd ID Out"=w722:T3)  [unwired: 3 in]
                n212 = call-poly <vilib>:"Start Motion.flx"("error in (no error)"=w720, "Axis or Vector Space"=w721, "Board ID"=w722) -> ()  [unwired: 3 in, 3 out]
              }
            }
            n213 = case shown="True" w649 {
              tunnel: w642 -> [_ w695]
              tunnel: w641 -> [_ w694]
              frame False {
              }
              frame True {
                w693 = T7 3 items=["Axis Control"=0, "Axis 1"=1, "Axis 2"=2, "Axis 3"=3, "Axis 4"=4, "Axis 5"=5, "Axis 6"=6, "Axis 7"=7, "Axis 8"=8, "Vector Space Control"=16, "Vector Space 1"=17, "Vector Space 2"=18, "Vector Space 3"=19, "Vector Space 4"=20] ("Axis or Vector Space")
                n214 = local read "Velocity (mm/s)"() -> (w702:dbl)
                n215 = local read "Multiplier"() -> (w696:dbl)
                n216 = Divide(x=w702, y=0.0125) -> (x/y=w698:dbl)
                n217 = Multiply(x=w698, y=w696) -> (x*y=w697:dbl)
                n218 = call <vilib>:"Set Operation Mode.flx"("Position Mode (Absolute)"=T4."Velocity", "error in (no error)"=w694, "Axis or Vector Space"=w693, "Board ID"=w695) -> ("error out"=w690:errorcluster, "Resource Output"=w692:T8, "Bd ID Out"=w691:T3)  [unwired: 2 in]
                n219 = To Long Integer(number=w697) -> (32bit integer=w701:i32)
                n220 = Multiply(x=w701, y=-1) -> (x*y=w699:i32)
                n221 = call <vilib>:"Load Velocity.flx"("Velocity (10000)"=w699, "error in (no error)"=w690, "Axis or Vector Space"=w692, "Board ID"=w691) -> ("error out"=w704:errorcluster, "Resource Output"=w705:T8, "Bd ID Out"=w706:T3)  [unwired: 3 in]
                n222 = call-poly <vilib>:"Start Motion.flx"("error in (no error)"=w704, "Axis or Vector Space"=w705, "Board ID"=w706) -> ()  [unwired: 3 in, 3 out]
              }
            }
          }
          event Key Up {
            n223 = event-data() -> ("ScanCode"=w758:i16)  [unwired: 1 in, 7 out]
            n224 = Equal?(x=i16 75, y=w758) -> (x = y?=w768:bool)
            n225 = Equal?(x=i16 77, y=w758) -> (x = y?=w766:bool)
            n226 = Equal?(x=i16 73, y=w758) -> (x = y?=w763:bool)
            n227 = Equal?(x=i16 81, y=w758) -> (x = y?=w761:bool)
            n228 = Equal?(x=i16 72, y=w758) -> (x = y?=w773:bool)
            n229 = Equal?(x=i16 80, y=w758) -> (x = y?=w771:bool)
            n230 = Or(x=w768, y=w766) -> (x .or. y?=w765:bool)
            n231 = Or(x=w763, y=w761) -> (x .or. y?=w760:bool)
            n232 = Or(x=w773, y=w771) -> (x .or. y?=w770:bool)
            n233 = case shown="True" w770 {
              tunnel: w757 -> [_ w783]
              tunnel: w759 -> [_ w781]
              frame False {
              }
              frame True {
                w782 = T7 2 items=["Axis Control"=0, "Axis 1"=1, "Axis 2"=2, "Axis 3"=3, "Axis 4"=4, "Axis 5"=5, "Axis 6"=6, "Axis 7"=7, "Axis 8"=8, "Vector Space Control"=16, "Vector Space 1"=17, "Vector Space 2"=18, "Vector Space 3"=19, "Vector Space 4"=20] ("Axis or Vector Space")
                n234 = call-poly <vilib>:"Stop Motion.flx"("error in (no error)"=w781, "Axis or Vector Space"=w782, "Board ID"=w783) -> ()  [unwired: 4 in, 3 out]
              }
            }
            n235 = case shown="True" w765 {
              tunnel: w757 -> [_ w780]
              tunnel: w759 -> [_ w778]
              frame False {
              }
              frame True {
                w779 = T7 3 items=["Axis Control"=0, "Axis 1"=1, "Axis 2"=2, "Axis 3"=3, "Axis 4"=4, "Axis 5"=5, "Axis 6"=6, "Axis 7"=7, "Axis 8"=8, "Vector Space Control"=16, "Vector Space 1"=17, "Vector Space 2"=18, "Vector Space 3"=19, "Vector Space 4"=20] ("Axis or Vector Space")
                n236 = call-poly <vilib>:"Stop Motion.flx"("error in (no error)"=w778, "Axis or Vector Space"=w779, "Board ID"=w780) -> ()  [unwired: 4 in, 3 out]
              }
            }
            n237 = case shown="True" w760 {
              tunnel: w757 -> [_ w777]
              tunnel: w759 -> [_ w775]
              frame False {
              }
              frame True {
                w776 = T7 4 items=["Axis Control"=0, "Axis 1"=1, "Axis 2"=2, "Axis 3"=3, "Axis 4"=4, "Axis 5"=5, "Axis 6"=6, "Axis 7"=7, "Axis 8"=8, "Vector Space Control"=16, "Vector Space 1"=17, "Vector Space 2"=18, "Vector Space 3"=19, "Vector Space 4"=20] ("Axis or Vector Space")
                n238 = call-poly <vilib>:"Stop Motion.flx"("error in (no error)"=w775, "Axis or Vector Space"=w776, "Board ID"=w777) -> ()  [unwired: 4 in, 3 out]
              }
            }
          }
        }
        n239 = event shown="[4] \"Jog Down\": Value Change" {
          selector: _ -> [_ _ _ _ _ _ _]
          dyn-events: _ -> [_ _ _ _ _ _ _]
          timeout: 0 -> [_ _ _ _ _ _ _]
          tunnel: w443 -> [_ w786 w808 w830 w852 w876 w900]
          tunnel: w442 -> [_ w785 w807 w829 w851 w875 w899]
          event Timeout {
            n240 = event-data() -> ()  [unwired: 1 in, 3 out]
          }
          event "Jog Up": Value Change {
            n241 = event-data() -> ("NewVal"=w784:bool)  [unwired: 1 in, 5 out]
            n242 = case shown="True" w784 {
              tunnel: w786 -> [w788 w794]
              tunnel: w785 -> [w787 w793]
              frame False {
                w789 = T7 2 items=["Axis Control"=0, "Axis 1"=1, "Axis 2"=2, "Axis 3"=3, "Axis 4"=4, "Axis 5"=5, "Axis 6"=6, "Axis 7"=7, "Axis 8"=8, "Vector Space Control"=16, "Vector Space 1"=17, "Vector Space 2"=18, "Vector Space 3"=19, "Vector Space 4"=20] ("Axis or Vector Space")
                n243 = call-poly <vilib>:"Stop Motion.flx"("error in (no error)"=w787, "Axis or Vector Space"=w789, "Board ID"=w788) -> ()  [unwired: 4 in, 3 out]
              }
              frame True {
                w798 = T7 2 items=["Axis Control"=0, "Axis 1"=1, "Axis 2"=2, "Axis 3"=3, "Axis 4"=4, "Axis 5"=5, "Axis 6"=6, "Axis 7"=7, "Axis 8"=8, "Vector Space Control"=16, "Vector Space 1"=17, "Vector Space 2"=18, "Vector Space 3"=19, "Vector Space 4"=20] ("Axis or Vector Space")
                n244 = local read "Velocity (mm/s)"() -> (w791:dbl)
                n245 = local read "Multiplier"() -> (w790:dbl)
                n246 = Divide(x=w791, y=0.0125) -> (x/y=w800:dbl)
                n247 = Multiply(x=w800, y=w790) -> (x*y=w799:dbl)
                n248 = call <vilib>:"Set Operation Mode.flx"("Position Mode (Absolute)"=T4."Velocity", "error in (no error)"=w793, "Axis or Vector Space"=w798, "Board ID"=w794) -> ("error out"=w795:errorcluster, "Resource Output"=w796:T8, "Bd ID Out"=w797:T3)  [unwired: 2 in]
                n249 = To Long Integer(number=w799) -> (32bit integer=w801:i32)
                n250 = call <vilib>:"Load Velocity.flx"("Velocity (10000)"=w801, "error in (no error)"=w795, "Axis or Vector Space"=w796, "Board ID"=w797) -> ("error out"=w803:errorcluster, "Resource Output"=w804:T8, "Bd ID Out"=w805:T3)  [unwired: 3 in]
                n251 = call-poly <vilib>:"Start Motion.flx"("error in (no error)"=w803, "Axis or Vector Space"=w804, "Board ID"=w805) -> ()  [unwired: 3 in, 3 out]
              }
            }
          }
          event "Jog Right": Value Change {
            n252 = event-data() -> ("NewVal"=w806:bool)  [unwired: 1 in, 5 out]
            n253 = case shown="True" w806 {
              tunnel: w808 -> [w810 w816]
              tunnel: w807 -> [w809 w815]
              frame False {
                w811 = T7 3 items=["Axis Control"=0, "Axis 1"=1, "Axis 2"=2, "Axis 3"=3, "Axis 4"=4, "Axis 5"=5, "Axis 6"=6, "Axis 7"=7, "Axis 8"=8, "Vector Space Control"=16, "Vector Space 1"=17, "Vector Space 2"=18, "Vector Space 3"=19, "Vector Space 4"=20] ("Axis or Vector Space")
                n254 = call-poly <vilib>:"Stop Motion.flx"("error in (no error)"=w809, "Axis or Vector Space"=w811, "Board ID"=w810) -> ()  [unwired: 4 in, 3 out]
              }
              frame True {
                w820 = T7 3 items=["Axis Control"=0, "Axis 1"=1, "Axis 2"=2, "Axis 3"=3, "Axis 4"=4, "Axis 5"=5, "Axis 6"=6, "Axis 7"=7, "Axis 8"=8, "Vector Space Control"=16, "Vector Space 1"=17, "Vector Space 2"=18, "Vector Space 3"=19, "Vector Space 4"=20] ("Axis or Vector Space")
                n255 = local read "Velocity (mm/s)"() -> (w813:dbl)
                n256 = local read "Multiplier"() -> (w812:dbl)
                n257 = Divide(x=w813, y=0.0125) -> (x/y=w822:dbl)
                n258 = Multiply(x=w822, y=w812) -> (x*y=w821:dbl)
                n259 = call <vilib>:"Set Operation Mode.flx"("Position Mode (Absolute)"=T4."Velocity", "error in (no error)"=w815, "Axis or Vector Space"=w820, "Board ID"=w816) -> ("error out"=w817:errorcluster, "Resource Output"=w818:T8, "Bd ID Out"=w819:T3)  [unwired: 2 in]
                n260 = To Long Integer(number=w821) -> (32bit integer=w823:i32)
                n261 = call <vilib>:"Load Velocity.flx"("Velocity (10000)"=w823, "error in (no error)"=w817, "Axis or Vector Space"=w818, "Board ID"=w819) -> ("error out"=w825:errorcluster, "Resource Output"=w826:T8, "Bd ID Out"=w827:T3)  [unwired: 3 in]
                n262 = call-poly <vilib>:"Start Motion.flx"("error in (no error)"=w825, "Axis or Vector Space"=w826, "Board ID"=w827) -> ()  [unwired: 3 in, 3 out]
              }
            }
          }
          event "Jog Far": Value Change {
            n263 = event-data() -> ("NewVal"=w828:bool)  [unwired: 1 in, 5 out]
            n264 = case shown="True" w828 {
              tunnel: w830 -> [w832 w838]
              tunnel: w829 -> [w831 w837]
              frame False {
                w833 = T7 4 items=["Axis Control"=0, "Axis 1"=1, "Axis 2"=2, "Axis 3"=3, "Axis 4"=4, "Axis 5"=5, "Axis 6"=6, "Axis 7"=7, "Axis 8"=8, "Vector Space Control"=16, "Vector Space 1"=17, "Vector Space 2"=18, "Vector Space 3"=19, "Vector Space 4"=20] ("Axis or Vector Space")
                n265 = call-poly <vilib>:"Stop Motion.flx"("error in (no error)"=w831, "Axis or Vector Space"=w833, "Board ID"=w832) -> ()  [unwired: 4 in, 3 out]
              }
              frame True {
                w842 = T7 4 items=["Axis Control"=0, "Axis 1"=1, "Axis 2"=2, "Axis 3"=3, "Axis 4"=4, "Axis 5"=5, "Axis 6"=6, "Axis 7"=7, "Axis 8"=8, "Vector Space Control"=16, "Vector Space 1"=17, "Vector Space 2"=18, "Vector Space 3"=19, "Vector Space 4"=20] ("Axis or Vector Space")
                n266 = local read "Velocity (mm/s)"() -> (w835:dbl)
                n267 = local read "Multiplier"() -> (w834:dbl)
                n268 = Divide(x=w835, y=0.0125) -> (x/y=w844:dbl)
                n269 = Multiply(x=w844, y=w834) -> (x*y=w843:dbl)
                n270 = call <vilib>:"Set Operation Mode.flx"("Position Mode (Absolute)"=T4."Velocity", "error in (no error)"=w837, "Axis or Vector Space"=w842, "Board ID"=w838) -> ("error out"=w839:errorcluster, "Resource Output"=w840:T8, "Bd ID Out"=w841:T3)  [unwired: 2 in]
                n271 = To Long Integer(number=w843) -> (32bit integer=w845:i32)
                n272 = call <vilib>:"Load Velocity.flx"("Velocity (10000)"=w845, "error in (no error)"=w839, "Axis or Vector Space"=w840, "Board ID"=w841) -> ("error out"=w847:errorcluster, "Resource Output"=w848:T8, "Bd ID Out"=w849:T3)  [unwired: 3 in]
                n273 = call-poly <vilib>:"Start Motion.flx"("error in (no error)"=w847, "Axis or Vector Space"=w848, "Board ID"=w849) -> ()  [unwired: 3 in, 3 out]
              }
            }
          }
          event "Jog Down": Value Change {
            n274 = event-data() -> ("NewVal"=w850:bool)  [unwired: 1 in, 5 out]
            n275 = case shown="True" w850 {
              tunnel: w852 -> [w854 w863]
              tunnel: w851 -> [w853 w862]
              frame False {
                w855 = T7 2 items=["Axis Control"=0, "Axis 1"=1, "Axis 2"=2, "Axis 3"=3, "Axis 4"=4, "Axis 5"=5, "Axis 6"=6, "Axis 7"=7, "Axis 8"=8, "Vector Space Control"=16, "Vector Space 1"=17, "Vector Space 2"=18, "Vector Space 3"=19, "Vector Space 4"=20] ("Axis or Vector Space")
                n276 = call-poly <vilib>:"Stop Motion.flx"("error in (no error)"=w853, "Axis or Vector Space"=w855, "Board ID"=w854) -> ()  [unwired: 4 in, 3 out]
              }
              frame True {
                w867 = T7 2 items=["Axis Control"=0, "Axis 1"=1, "Axis 2"=2, "Axis 3"=3, "Axis 4"=4, "Axis 5"=5, "Axis 6"=6, "Axis 7"=7, "Axis 8"=8, "Vector Space Control"=16, "Vector Space 1"=17, "Vector Space 2"=18, "Vector Space 3"=19, "Vector Space 4"=20] ("Axis or Vector Space")
                n277 = local read "Velocity (mm/s)"() -> (w860:dbl)
                n278 = local read "Multiplier"() -> (w859:dbl)
                n279 = Divide(x=w860, y=0.0125) -> (x/y=w869:dbl)
                n280 = Multiply(x=w869, y=w859) -> (x*y=w868:dbl)
                n281 = call <vilib>:"Set Operation Mode.flx"("Position Mode (Absolute)"=T4."Velocity", "error in (no error)"=w862, "Axis or Vector Space"=w867, "Board ID"=w863) -> ("error out"=w864:errorcluster, "Resource Output"=w865:T8, "Bd ID Out"=w866:T3)  [unwired: 2 in]
                n282 = To Long Integer(number=w868) -> (32bit integer=w858:i32)
                n283 = Multiply(x=w858, y=-1) -> (x*y=w857:i32)
                n284 = call <vilib>:"Load Velocity.flx"("Velocity (10000)"=w857, "error in (no error)"=w864, "Axis or Vector Space"=w865, "Board ID"=w866) -> ("error out"=w871:errorcluster, "Resource Output"=w872:T8, "Bd ID Out"=w873:T3)  [unwired: 3 in]
                n285 = call-poly <vilib>:"Start Motion.flx"("error in (no error)"=w871, "Axis or Vector Space"=w872, "Board ID"=w873) -> ()  [unwired: 3 in, 3 out]
              }
            }
          }
          event "Jog Left": Value Change {
            n286 = event-data() -> ("NewVal"=w874:bool)  [unwired: 1 in, 5 out]
            n287 = case shown="True" w874 {
              tunnel: w876 -> [w878 w887]
              tunnel: w875 -> [w877 w886]
              frame False {
                w879 = T7 3 items=["Axis Control"=0, "Axis 1"=1, "Axis 2"=2, "Axis 3"=3, "Axis 4"=4, "Axis 5"=5, "Axis 6"=6, "Axis 7"=7, "Axis 8"=8, "Vector Space Control"=16, "Vector Space 1"=17, "Vector Space 2"=18, "Vector Space 3"=19, "Vector Space 4"=20] ("Axis or Vector Space")
                n288 = call-poly <vilib>:"Stop Motion.flx"("error in (no error)"=w877, "Axis or Vector Space"=w879, "Board ID"=w878) -> ()  [unwired: 4 in, 3 out]
              }
              frame True {
                w891 = T7 3 items=["Axis Control"=0, "Axis 1"=1, "Axis 2"=2, "Axis 3"=3, "Axis 4"=4, "Axis 5"=5, "Axis 6"=6, "Axis 7"=7, "Axis 8"=8, "Vector Space Control"=16, "Vector Space 1"=17, "Vector Space 2"=18, "Vector Space 3"=19, "Vector Space 4"=20] ("Axis or Vector Space")
                n289 = local read "Velocity (mm/s)"() -> (w884:dbl)
                n290 = local read "Multiplier"() -> (w883:dbl)
                n291 = Divide(x=w884, y=0.0125) -> (x/y=w893:dbl)
                n292 = Multiply(x=w893, y=w883) -> (x*y=w892:dbl)
                n293 = call <vilib>:"Set Operation Mode.flx"("Position Mode (Absolute)"=T4."Velocity", "error in (no error)"=w886, "Axis or Vector Space"=w891, "Board ID"=w887) -> ("error out"=w888:errorcluster, "Resource Output"=w889:T8, "Bd ID Out"=w890:T3)  [unwired: 2 in]
                n294 = To Long Integer(number=w892) -> (32bit integer=w882:i32)
                n295 = Multiply(x=w882, y=-1) -> (x*y=w881:i32)
                n296 = call <vilib>:"Load Velocity.flx"("Velocity (10000)"=w881, "error in (no error)"=w888, "Axis or Vector Space"=w889, "Board ID"=w890) -> ("error out"=w895:errorcluster, "Resource Output"=w896:T8, "Bd ID Out"=w897:T3)  [unwired: 3 in]
                n297 = call-poly <vilib>:"Start Motion.flx"("error in (no error)"=w895, "Axis or Vector Space"=w896, "Board ID"=w897) -> ()  [unwired: 3 in, 3 out]
              }
            }
          }
          event "Jog Close": Value Change {
            n298 = event-data() -> ("NewVal"=w898:bool)  [unwired: 1 in, 5 out]
            n299 = case shown="True" w898 {
              tunnel: w900 -> [w902 w911]
              tunnel: w899 -> [w901 w910]
              frame False {
                w903 = T7 4 items=["Axis Control"=0, "Axis 1"=1, "Axis 2"=2, "Axis 3"=3, "Axis 4"=4, "Axis 5"=5, "Axis 6"=6, "Axis 7"=7, "Axis 8"=8, "Vector Space Control"=16, "Vector Space 1"=17, "Vector Space 2"=18, "Vector Space 3"=19, "Vector Space 4"=20] ("Axis or Vector Space")
                n300 = call-poly <vilib>:"Stop Motion.flx"("error in (no error)"=w901, "Axis or Vector Space"=w903, "Board ID"=w902) -> ()  [unwired: 4 in, 3 out]
              }
              frame True {
                w915 = T7 4 items=["Axis Control"=0, "Axis 1"=1, "Axis 2"=2, "Axis 3"=3, "Axis 4"=4, "Axis 5"=5, "Axis 6"=6, "Axis 7"=7, "Axis 8"=8, "Vector Space Control"=16, "Vector Space 1"=17, "Vector Space 2"=18, "Vector Space 3"=19, "Vector Space 4"=20] ("Axis or Vector Space")
                n301 = local read "Velocity (mm/s)"() -> (w908:dbl)
                n302 = local read "Multiplier"() -> (w907:dbl)
                n303 = Divide(x=w908, y=0.0125) -> (x/y=w917:dbl)
                n304 = Multiply(x=w917, y=w907) -> (x*y=w916:dbl)
                n305 = call <vilib>:"Set Operation Mode.flx"("Position Mode (Absolute)"=T4."Velocity", "error in (no error)"=w910, "Axis or Vector Space"=w915, "Board ID"=w911) -> ("error out"=w912:errorcluster, "Resource Output"=w913:T8, "Bd ID Out"=w914:T3)  [unwired: 2 in]
                n306 = To Long Integer(number=w916) -> (32bit integer=w906:i32)
                n307 = Multiply(x=w906, y=-1) -> (x*y=w905:i32)
                n308 = call <vilib>:"Load Velocity.flx"("Velocity (10000)"=w905, "error in (no error)"=w912, "Axis or Vector Space"=w913, "Board ID"=w914) -> ("error out"=w919:errorcluster, "Resource Output"=w920:T8, "Bd ID Out"=w921:T3)  [unwired: 3 in]
                n309 = call-poly <vilib>:"Start Motion.flx"("error in (no error)"=w919, "Axis or Vector Space"=w920, "Board ID"=w921) -> ()  [unwired: 3 in, 3 out]
              }
            }
          }
        }
        n310 = event shown="[6] \"Move Close\": Value Change" {
          selector: _ -> [_ _ _ _ _ _ _]
          dyn-events: _ -> [_ _ _ _ _ _ _]
          timeout: 0 -> [_ _ _ _ _ _ _]
          tunnel: w443 -> [_ w497 w520 w543 w566 w591 w616]
          tunnel: w442 -> [_ w496 w519 w542 w565 w590 w615]
          event Timeout {
            n311 = event-data() -> ()  [unwired: 1 in, 3 out]
          }
          event "Move Up": Value Change {
            n312 = event-data() -> ("NewVal"=w498:bool)  [unwired: 1 in, 5 out]
            n313 = case shown="True" w498 {
              tunnel: w497 -> [_ w507]
              tunnel: w496 -> [_ w508]
              frame False {
              }
              frame True {
                w501 = 0.0125 ("y")
                w503 = T7 2 items=["Axis Control"=0, "Axis 1"=1, "Axis 2"=2, "Axis 3"=3, "Axis 4"=4, "Axis 5"=5, "Axis 6"=6, "Axis 7"=7, "Axis 8"=8, "Vector Space Control"=16, "Vector Space 1"=17, "Vector Space 2"=18, "Vector Space 3"=19, "Vector Space 4"=20] ("Axis or Vector Space")
                n314 = local read "Move (mm)"() -> (w511:dbl)
                n315 = local read "Velocity (mm/s)"() -> (w502:dbl)
                n316 = Divide(x=w511, y=w501) -> (x/y=w510:dbl)
                n317 = Divide(x=w502, y=w501) -> (x/y=w500:dbl)
                n318 = To Long Integer(number=w500) -> (32bit integer=w499:i32)
                n319 = To Long Integer(number=w510) -> (32bit integer=w509:i32)
                n320 = call <vilib>:"Load Velocity.flx"("Velocity (10000)"=w499, "error in (no error)"=w508, "Axis or Vector Space"=w503, "Board ID"=w507) -> ("error out"=w505:errorcluster, "Resource Output"=w504:T8, "Bd ID Out"=w506:T3)  [unwired: 3 in]
                n321 = call <vilib>:"Set Operation Mode.flx"("Position Mode (Absolute)"=T4."Relative Position", "error in (no error)"=w505, "Axis or Vector Space"=w504, "Board ID"=w506) -> ("error out"=w514:errorcluster, "Resource Output"=w515:T8, "Bd ID Out"=w516:T3)  [unwired: 2 in]
                n322 = call <vilib>:"Load Target Position.flx"("Target Position (0)"=w509, "error in (no error)"=w514, "Axis"=w515, "Board ID"=w516) -> ("error out"=w517:errorcluster, "Resource Output"=w512:T8, "Bd ID Out"=w513:T3)  [unwired: 3 in]
                n323 = call-poly <vilib>:"Start Motion.flx"("error in (no error)"=w517, "Axis or Vector Space"=w512, "Board ID"=w513) -> ()  [unwired: 3 in, 3 out]
              }
            }
          }
          event "Move Right": Value Change {
            n324 = event-data() -> ("NewVal"=w521:bool)  [unwired: 1 in, 5 out]
            n325 = case shown="True" w521 {
              tunnel: w520 -> [_ w530]
              tunnel: w519 -> [_ w531]
              frame False {
              }
              frame True {
                w524 = 0.0125 ("y")
                w526 = T7 3 items=["Axis Control"=0, "Axis 1"=1, "Axis 2"=2, "Axis 3"=3, "Axis 4"=4, "Axis 5"=5, "Axis 6"=6, "Axis 7"=7, "Axis 8"=8, "Vector Space Control"=16, "Vector Space 1"=17, "Vector Space 2"=18, "Vector Space 3"=19, "Vector Space 4"=20] ("Axis or Vector Space")
                n326 = local read "Move (mm)"() -> (w534:dbl)
                n327 = local read "Velocity (mm/s)"() -> (w525:dbl)
                n328 = Divide(x=w534, y=w524) -> (x/y=w533:dbl)
                n329 = Divide(x=w525, y=w524) -> (x/y=w523:dbl)
                n330 = To Long Integer(number=w523) -> (32bit integer=w522:i32)
                n331 = To Long Integer(number=w533) -> (32bit integer=w532:i32)
                n332 = call <vilib>:"Load Velocity.flx"("Velocity (10000)"=w522, "error in (no error)"=w531, "Axis or Vector Space"=w526, "Board ID"=w530) -> ("error out"=w528:errorcluster, "Resource Output"=w527:T8, "Bd ID Out"=w529:T3)  [unwired: 3 in]
                n333 = call <vilib>:"Set Operation Mode.flx"("Position Mode (Absolute)"=T4."Relative Position", "error in (no error)"=w528, "Axis or Vector Space"=w527, "Board ID"=w529) -> ("error out"=w537:errorcluster, "Resource Output"=w538:T8, "Bd ID Out"=w539:T3)  [unwired: 2 in]
                n334 = call <vilib>:"Load Target Position.flx"("Target Position (0)"=w532, "error in (no error)"=w537, "Axis"=w538, "Board ID"=w539) -> ("error out"=w540:errorcluster, "Resource Output"=w535:T8, "Bd ID Out"=w536:T3)  [unwired: 3 in]
                n335 = call-poly <vilib>:"Start Motion.flx"("error in (no error)"=w540, "Axis or Vector Space"=w535, "Board ID"=w536) -> ()  [unwired: 3 in, 3 out]
              }
            }
          }
          event "Move Far": Value Change {
            n336 = event-data() -> ("NewVal"=w544:bool)  [unwired: 1 in, 5 out]
            n337 = case shown="True" w544 {
              tunnel: w543 -> [_ w553]
              tunnel: w542 -> [_ w554]
              frame False {
              }
              frame True {
                w547 = 0.0125 ("y")
                w549 = T7 4 items=["Axis Control"=0, "Axis 1"=1, "Axis 2"=2, "Axis 3"=3, "Axis 4"=4, "Axis 5"=5, "Axis 6"=6, "Axis 7"=7, "Axis 8"=8, "Vector Space Control"=16, "Vector Space 1"=17, "Vector Space 2"=18, "Vector Space 3"=19, "Vector Space 4"=20] ("Axis or Vector Space")
                n338 = local read "Move (mm)"() -> (w557:dbl)
                n339 = local read "Velocity (mm/s)"() -> (w548:dbl)
                n340 = Divide(x=w557, y=w547) -> (x/y=w556:dbl)
                n341 = Divide(x=w548, y=w547) -> (x/y=w546:dbl)
                n342 = To Long Integer(number=w546) -> (32bit integer=w545:i32)
                n343 = To Long Integer(number=w556) -> (32bit integer=w555:i32)
                n344 = call <vilib>:"Load Velocity.flx"("Velocity (10000)"=w545, "error in (no error)"=w554, "Axis or Vector Space"=w549, "Board ID"=w553) -> ("error out"=w551:errorcluster, "Resource Output"=w550:T8, "Bd ID Out"=w552:T3)  [unwired: 3 in]
                n345 = call <vilib>:"Set Operation Mode.flx"("Position Mode (Absolute)"=T4."Relative Position", "error in (no error)"=w551, "Axis or Vector Space"=w550, "Board ID"=w552) -> ("error out"=w560:errorcluster, "Resource Output"=w561:T8, "Bd ID Out"=w562:T3)  [unwired: 2 in]
                n346 = call <vilib>:"Load Target Position.flx"("Target Position (0)"=w555, "error in (no error)"=w560, "Axis"=w561, "Board ID"=w562) -> ("error out"=w563:errorcluster, "Resource Output"=w558:T8, "Bd ID Out"=w559:T3)  [unwired: 3 in]
                n347 = call-poly <vilib>:"Start Motion.flx"("error in (no error)"=w563, "Axis or Vector Space"=w558, "Board ID"=w559) -> ()  [unwired: 3 in, 3 out]
              }
            }
          }
          event "Move Down": Value Change {
            n348 = event-data() -> ("NewVal"=w567:bool)  [unwired: 1 in, 5 out]
            n349 = case shown="True" w567 {
              tunnel: w566 -> [_ w579]
              tunnel: w565 -> [_ w580]
              frame False {
              }
              frame True {
                w573 = 0.0125 ("y")
                w575 = T7 2 items=["Axis Control"=0, "Axis 1"=1, "Axis 2"=2, "Axis 3"=3, "Axis 4"=4, "Axis 5"=5, "Axis 6"=6, "Axis 7"=7, "Axis 8"=8, "Vector Space Control"=16, "Vector Space 1"=17, "Vector Space 2"=18, "Vector Space 3"=19, "Vector Space 4"=20] ("Axis or Vector Space")
                n350 = local read "Move (mm)"() -> (w582:dbl)
                n351 = local read "Velocity (mm/s)"() -> (w574:dbl)
                n352 = Divide(x=w582, y=w573) -> (x/y=w581:dbl)
                n353 = Divide(x=w574, y=w573) -> (x/y=w572:dbl)
                n354 = To Long Integer(number=w572) -> (32bit integer=w571:i32)
                n355 = To Long Integer(number=w581) -> (32bit integer=w570:i32)
                n356 = call <vilib>:"Load Velocity.flx"("Velocity (10000)"=w571, "error in (no error)"=w580, "Axis or Vector Space"=w575, "Board ID"=w579) -> ("error out"=w577:errorcluster, "Resource Output"=w576:T8, "Bd ID Out"=w578:T3)  [unwired: 3 in]
                n357 = call <vilib>:"Set Operation Mode.flx"("Position Mode (Absolute)"=T4."Relative Position", "error in (no error)"=w577, "Axis or Vector Space"=w576, "Board ID"=w578) -> ("error out"=w585:errorcluster, "Resource Output"=w586:T8, "Bd ID Out"=w587:T3)  [unwired: 2 in]
                n358 = Multiply(x=w570, y=-1) -> (x*y=w569:i32)
                n359 = call <vilib>:"Load Target Position.flx"("Target Position (0)"=w569, "error in (no error)"=w585, "Axis"=w586, "Board ID"=w587) -> ("error out"=w588:errorcluster, "Resource Output"=w583:T8, "Bd ID Out"=w584:T3)  [unwired: 3 in]
                n360 = call-poly <vilib>:"Start Motion.flx"("error in (no error)"=w588, "Axis or Vector Space"=w583, "Board ID"=w584) -> ()  [unwired: 3 in, 3 out]
              }
            }
          }
          event "Move Left": Value Change {
            n361 = event-data() -> ("NewVal"=w592:bool)  [unwired: 1 in, 5 out]
            n362 = case shown="True" w592 {
              tunnel: w591 -> [_ w604]
              tunnel: w590 -> [_ w605]
              frame False {
              }
              frame True {
                w598 = 0.0125 ("y")
                w600 = T7 3 items=["Axis Control"=0, "Axis 1"=1, "Axis 2"=2, "Axis 3"=3, "Axis 4"=4, "Axis 5"=5, "Axis 6"=6, "Axis 7"=7, "Axis 8"=8, "Vector Space Control"=16, "Vector Space 1"=17, "Vector Space 2"=18, "Vector Space 3"=19, "Vector Space 4"=20] ("Axis or Vector Space")
                n363 = local read "Move (mm)"() -> (w607:dbl)
                n364 = local read "Velocity (mm/s)"() -> (w599:dbl)
                n365 = Divide(x=w607, y=w598) -> (x/y=w606:dbl)
                n366 = Divide(x=w599, y=w598) -> (x/y=w597:dbl)
                n367 = To Long Integer(number=w597) -> (32bit integer=w596:i32)
                n368 = To Long Integer(number=w606) -> (32bit integer=w595:i32)
                n369 = call <vilib>:"Load Velocity.flx"("Velocity (10000)"=w596, "error in (no error)"=w605, "Axis or Vector Space"=w600, "Board ID"=w604) -> ("error out"=w602:errorcluster, "Resource Output"=w601:T8, "Bd ID Out"=w603:T3)  [unwired: 3 in]
                n370 = call <vilib>:"Set Operation Mode.flx"("Position Mode (Absolute)"=T4."Relative Position", "error in (no error)"=w602, "Axis or Vector Space"=w601, "Board ID"=w603) -> ("error out"=w610:errorcluster, "Resource Output"=w611:T8, "Bd ID Out"=w612:T3)  [unwired: 2 in]
                n371 = Multiply(x=w595, y=-1) -> (x*y=w594:i32)
                n372 = call <vilib>:"Load Target Position.flx"("Target Position (0)"=w594, "error in (no error)"=w610, "Axis"=w611, "Board ID"=w612) -> ("error out"=w613:errorcluster, "Resource Output"=w608:T8, "Bd ID Out"=w609:T3)  [unwired: 3 in]
                n373 = call-poly <vilib>:"Start Motion.flx"("error in (no error)"=w613, "Axis or Vector Space"=w608, "Board ID"=w609) -> ()  [unwired: 3 in, 3 out]
              }
            }
          }
          event "Move Close": Value Change {
            n374 = event-data() -> ("NewVal"=w617:bool)  [unwired: 1 in, 5 out]
            n375 = case shown="True" w617 {
              tunnel: w616 -> [_ w629]
              tunnel: w615 -> [_ w630]
              frame False {
              }
              frame True {
                w623 = 0.0125 ("y")
                w625 = T7 4 items=["Axis Control"=0, "Axis 1"=1, "Axis 2"=2, "Axis 3"=3, "Axis 4"=4, "Axis 5"=5, "Axis 6"=6, "Axis 7"=7, "Axis 8"=8, "Vector Space Control"=16, "Vector Space 1"=17, "Vector Space 2"=18, "Vector Space 3"=19, "Vector Space 4"=20] ("Axis or Vector Space")
                n376 = local read "Move (mm)"() -> (w632:dbl)
                n377 = local read "Velocity (mm/s)"() -> (w624:dbl)
                n378 = Divide(x=w632, y=w623) -> (x/y=w631:dbl)
                n379 = Divide(x=w624, y=w623) -> (x/y=w622:dbl)
                n380 = To Long Integer(number=w622) -> (32bit integer=w621:i32)
                n381 = To Long Integer(number=w631) -> (32bit integer=w620:i32)
                n382 = call <vilib>:"Load Velocity.flx"("Velocity (10000)"=w621, "error in (no error)"=w630, "Axis or Vector Space"=w625, "Board ID"=w629) -> ("error out"=w627:errorcluster, "Resource Output"=w626:T8, "Bd ID Out"=w628:T3)  [unwired: 3 in]
                n383 = call <vilib>:"Set Operation Mode.flx"("Position Mode (Absolute)"=T4."Relative Position", "error in (no error)"=w627, "Axis or Vector Space"=w626, "Board ID"=w628) -> ("error out"=w635:errorcluster, "Resource Output"=w636:T8, "Bd ID Out"=w637:T3)  [unwired: 2 in]
                n384 = Multiply(x=w620, y=-1) -> (x*y=w619:i32)
                n385 = call <vilib>:"Load Target Position.flx"("Target Position (0)"=w619, "error in (no error)"=w635, "Axis"=w636, "Board ID"=w637) -> ("error out"=w638:errorcluster, "Resource Output"=w633:T8, "Bd ID Out"=w634:T3)  [unwired: 3 in]
                n386 = call-poly <vilib>:"Start Motion.flx"("error in (no error)"=w638, "Axis or Vector Space"=w633, "Board ID"=w634) -> ()  [unwired: 3 in, 3 out]
              }
            }
          }
        }
        n387 = case shown="True" "Enable Oscilloscope" {
          tunnel: w440 -> [w448 w460]
          tunnel: w439 -> [w447 w461]
          tunnel: [w447 w472] -> w438
          tunnel: [w448 w471] -> w437
          frame False {
          }
          frame True {
            n388 = local read "trigger source"() -> (w458:T1)
            n389 = local read "trigger level"() -> (w459:dbl)
            n390 = local read "# Channel"() -> (w457:i32)
            n391 = local read "vertical offset"() -> (w455:dbl)
            n392 = local read "vertical range"() -> (w456:dbl)
            n393 = local read "Sample rate (MHz)"() -> (w454:dbl)
            n394 = local read "Time (us)"() -> (w453:dbl)
            n395 = call "config_Scope.vi"("instrument handle"=w461, "trigger source"=w458, "trigger level"=w459, "Channel"=w457, "vertical range"=w456, "vertical offset"=w455, "error in"=w460, "Frequency(MHz)"=w454, "Time(us)"=w453) -> ("instrument handle out"=w452:refnum<k15>, "Record length"=w449:i32, "Channel out"=w450:string, "error out"=w451:errorcluster)  [unwired: 3 in]
            n396 = local read "Pulses"() -> (w473:i32)
            n397 = call "mean_Scope.vi"("instrument handle in"=w452, "pulses"=w473, "channels"=w450, "record length"=w449, "error in"=w451) -> ("instrument handle out"=w472:refnum<k15>, "signal out"=w470:dbl[], "dt"=w466:dbl, "error out"=w471:errorcluster)  [unwired: 7 in]
            n398 = case shown="False" "Lowpass filter" {
              tunnel: w470 -> [w476 w495]
              tunnel: [w476 w492] -> w467
              tunnel: "Lowpass cut (kHz)" -> [_ w494]
              tunnel: "Highpass cut (kHz)" -> [_ w493]
              tunnel: w466 -> [w475 w490]
              frame False {
                n399 = Array Max & Min(array=w476) -> (max value=w489:dbl, max index (indices)=w484:i32, min value=w488:dbl)  [unwired: 1 out]
                n400 = Subtract(x=w489, y=w488) -> (x-y=w485:dbl)
                n401 = Multiply(x=w475, y=w484) -> (x*y=w477:dbl)
                n402 = Multiply(x=1000.0, y=w485) -> (x*y=w487:dbl)
                n403 = Multiply(x=1000000.0, y=w477) -> (x*y=→"Time (us)":dbl)
                n404 = Multiply(x=w477, y=1480.0) -> (x*y=w482:dbl)
                n405 = Multiply(x=w482, y=1000.0) -> (x*y=→"Distance (mm)":dbl)
                n406 = local write "Peak to peak"(w487) -> ()
              }
              frame True {
                n407 = call "bandpass_kHz.vi"("Highpass cut (kHz)"=w493, "Lowpass cut (kHz)"=w494, "dt"=w490, "Signal in"=w495) -> ("Peak2peak(mV)"=→"Peak to peak":dbl, "Signal out"=w492:dbl[])  [unwired: 6 in]
              }
            }
            n408 = call "WV_PS_graph.vi"("Power spectrum unit"="Power spectrum unit", "Time unit"="Time unit", "dt"=w466, "Signal in"=w467) -> ("Power Spectrum / PSD"=→"Frequency Graph":cluster{"f0":dbl, "df":dbl, "magnitude":dbl[]}, "output waveform"=→"Time Graph":waveform(dbl))  [unwired: 6 in]
          }
        }
        n409 = local read "Ajust Axis"() -> (w446:bool)
      }
      n410 = call <instrlib>:"niScope Close.vi"("instrument handle"=w431, "error in"=w430) -> ()  [unwired: 13 in, 1 out]
    }
  }
